vi "NF WF1973_74 CONS Toff.vi"(6 "Read(F)":bool, 7 "Time(0)":dbl min=0.0 max=20.0 step=0.01 format="%.2f", 8 "error in (no error)":errorcluster caption="Error IN", 9 "Set Time(Input)":u16(ring) items=["Input", "Minimum", "Maximum"], 10 "Ch(Ch1)":bool, 11 "VISAsession":refnum<visa-resource-name>) -> (0 "error out":errorcluster caption="Error OUT", 2 "Query Time":dbl=999.0 format="%.2f", 3 "CopyVISAsession":refnum<visa-resource-name>)   [LabVIEW 2010]
panel:
  # "Choose\nInput"
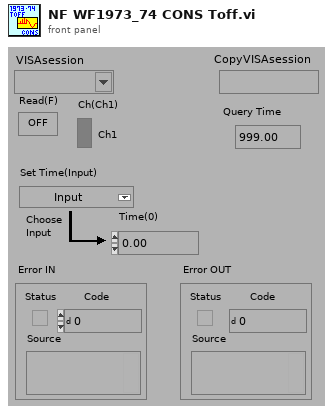
[diagram p1: front panel]
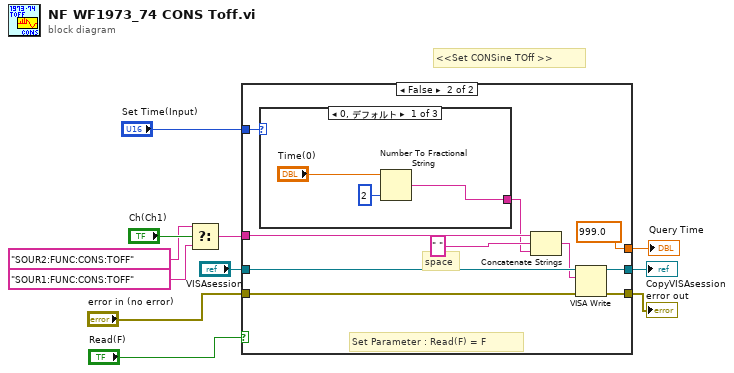
[diagram p0: block diagram]
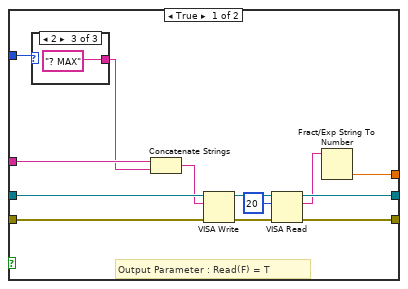
[diagram p2: hidden frame]
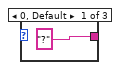
[diagram p3: hidden frame]
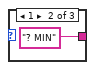
[diagram p4: hidden frame]
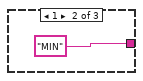
[diagram p5: hidden frame]
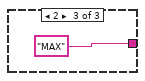
[diagram p6: hidden frame]
diagram:
  # "<<Set CONSine TOff >>"
  n1 = Select(t="SOUR2:FUNC:CONS:TOFF" ("文字列"), s="Ch(Ch1)", f="SOUR1:FUNC:CONS:TOFF" ("文字列")) -> (s? t:f=w4:string)
  n2 = case shown="FALSE" "Read(F)" {
    tunnel: "VISAsession" -> [w24 w37]
    tunnel: [w21 w35] -> w10
    tunnel: [w20 w36] -> w9
    tunnel: "error in (no error)" -> [w19 w31]
    tunnel: w4 -> [w17 w32]
    tunnel: [w14 999.0] -> w6
    tunnel: "Set Time(Input)" -> [w13 w30]
    frame True {
      # "Output Parameter : Read(F) = T"
      n3 = case shown="2" w13 {
        tunnel: ["?" ("形式文字列") "? MIN" ("形式文字列") "? MAX" ("形式文字列")] -> w12
        frame 0, Default {
        }
        frame 1 {
        }
        frame 2 {
        }
      }
      n4 = Concatenate Strings(w17, w12) -> (w16:string)
      n5 = VISA Write(VISA resource name=w24, write buffer=w16, error in (no error)=w19) -> (VISA resource name out=w22:refnum<visa-resource-name>, error out=w23:errorcluster)  [unwired: 1 out]
      n6 = VISA Read(VISA resource name=w22, byte count=u32 20 ("バイトカウント（0）"), error in (no error)=w23) -> (VISA resource name out=w21:refnum<visa-resource-name>, read buffer=w15:string, error out=w20:errorcluster)  [unwired: 1 out]
      n7 = Fract/Exp String To Number(string=w15) -> (number=w14:dbl)  [unwired: 3 in, 1 out]
    }
    frame False {
      # "space"
      # "Set Parameter : Read(F) = F"
      n8 = case shown="0, デフォルト" w30 {
        tunnel: [w39 "MIN" ("文字列") "MAX" ("文字列")] -> w29
        frame 0, Default {
          n9 = Number To Fractional String(number="Time(0)", precision (6)=i16 2 ("精度 (6)")) -> (F-format string=w39:string)  [unwired: 2 in]
        }
        frame 1 {
        }
        frame 2 {
        }
      }
      n10 = Concatenate Strings(w32, " ", w29) -> (w34:string)
      n11 = VISA Write(VISA resource name=w37, write buffer=w34, error in (no error)=w31) -> (VISA resource name out=w35:refnum<visa-resource-name>, error out=w36:errorcluster)  [unwired: 1 out]
    }
  }
  "error out" <- w9
  "CopyVISAsession" <- w10
  "Query Time" <- w6
